vi "StageSet.vi"(8 "error in (no error)":errorcluster, 11 "Microscope in":refnum<class "Microscope.lvclass">) -> (0 "error out":errorcluster, 3 "Microscope out":refnum<class "Microscope.lvclass">)   [LabVIEW 2012, in "Microscope.lvclass"]
uses:
  classes/Microscope.lvclass
  classes/Microscope.lvclass/Microscope.ctl
  variables/GlobalUI.vi
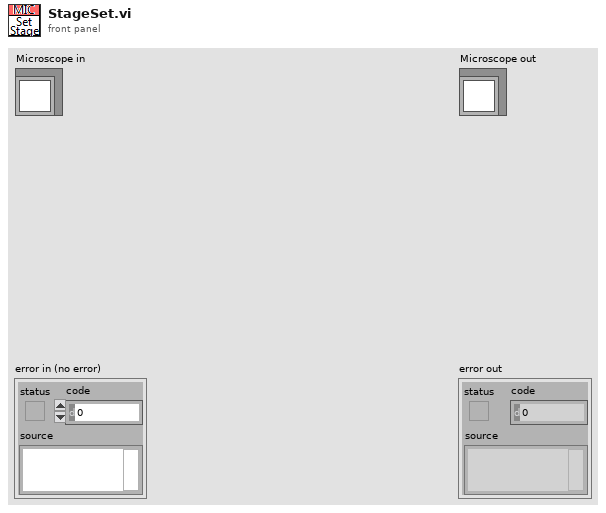
[diagram p1: front panel]
types:
  T1 = typedef "Move Type.ctl" = enum16{"None", "Continuous", "Discrete"}
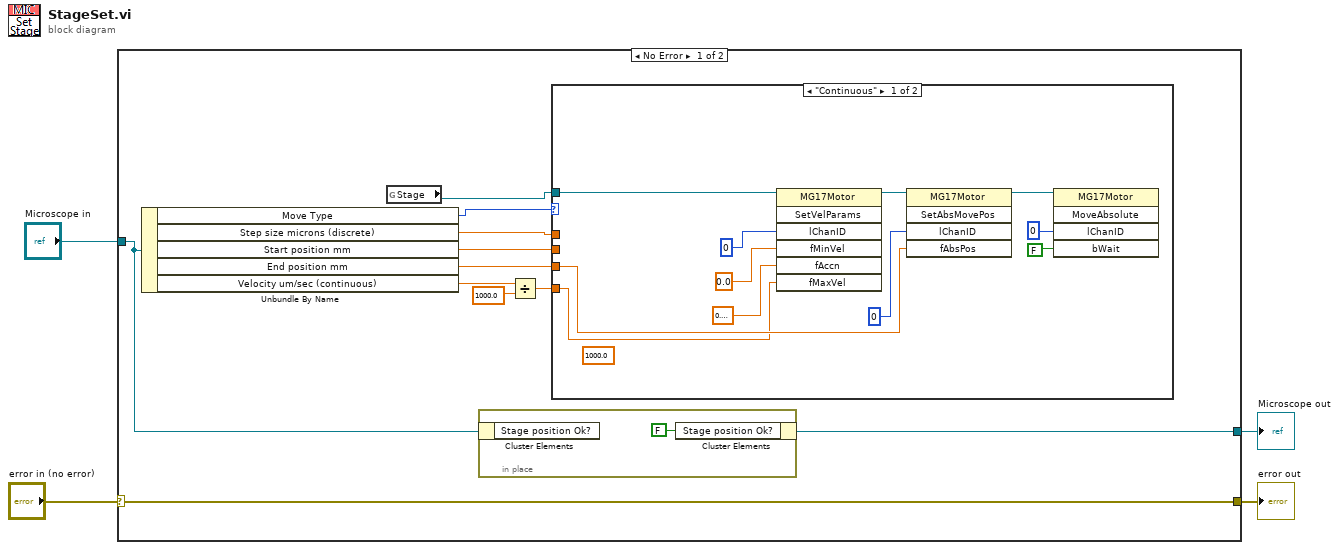
[diagram p0: block diagram]
diagram:
  n1 = case shown="No Error" "error in (no error)" {
    selector: "error in (no error)" -> [w15 w29]
    tunnel: [w15 w29] -> w3
    tunnel: [w7 w28] -> w1
    tunnel: "Microscope in" -> [w8 w28]
    frame No Error {
      n2 = Unbundle By Name(w8) -> ("Move Type"=w6:T1, "Step size microns (discrete)"=w12:dbl, "Start position mm"=w13:dbl, "End position mm"=w14:dbl, "Velocity um/sec (continuous)"=w10:dbl)
      n3 = global read "GlobalUI.vi" "Stage"() -> (w5:refnum<k7>)
      n4 = in-place {
        n5 = in-place-cluster #1(w8) -> ()  [unwired: 1 out]
        n6 = in-place-cluster #1("Stage position Ok?"=FALSE) -> (w7:refnum<class "Microscope.lvclass">)
      }
      n7 = Divide(x=w10, y=1000.0) -> (x/y=w9:dbl)
      n8 = case shown="\"Continuous\"" w6 {
        tunnel: w5 -> [w17 _]
        tunnel: w14 -> [w26 _]
        tunnel: w13 -> [_ _]
        tunnel: w12 -> [_ _]
        tunnel: w9 -> [w19 _]
        frame "Continuous" {
          (unwired) 1000.0 ("y")
          n9 = invoke class="MG17Motor" method="SetVelParams"(reference=w17, "lChanID"=0, "fMinVel"=sgl 0.0, "fAccn"=sgl 0.1, "fMaxVel"=w19) -> (reference out=w18:refnum<k7>)  [unwired: 2 in, 6 out]
          n10 = invoke class="MG17Motor" method="SetAbsMovePos"(reference=w18, "lChanID"=0, "fAbsPos"=w26) -> (reference out=w24:refnum<k7>)  [unwired: 2 in, 4 out]
          n11 = invoke class="MG17Motor" method="MoveAbsolute"(reference=w24, "lChanID"=0, "bWait"=FALSE) -> ()  [unwired: 2 in, 5 out]
        }
        frame "None", Default {
        }
      }
    }
    frame Error {
    }
  }
  "error out" <- w3
  "Microscope out" <- w1
